vi "3_dynamic_friction_main.vi"() -> ()   [LabVIEW 2019]
uses:
  Shared VIs/ENPID/PID_Settings.ctl
  Shared VIs/ENPID/Gains.ctl
  Shared VIs/ENPID/NonLinearGainParams.ctl
  Shared VIs/ENPID/NonLinearGain.ctl
  Shared VIs/ENPID/DPartVariable.ctl
  Shared VIs/ENPID/VelocityEstimate.ctl
  Shared VIs/ENPID/OutputRange.ctl
  Shared VIs/TypeDef_TDMS_States.ctl
  <vilib>/myRIO/Common/Instrument Driver Framework/myRIO v1.0/Encoder/typedefs/Encoder Signal Mode.ctl
  Shared VIs/ModelSpecific/ETHMikeModel.ctl
  Shared VIs/ModelSpecific/ReadOnlyGlobalActions.ctl
  <vilib>/myRIO/Instrument Drivers/Onboard IO/AI/typedefs/AI Reference.ctl
  <vilib>/myRIO/Common/Instrument Driver Framework/Utilities/typedefs/myRIO Generic Hardware Reference.ctl
  <vilib>/myRIO/Common/Instrument Driver Framework/Utilities/typedefs/Hardware Version Enum.ctl
  <vilib>/myRIO/Common/Instrument Driver Framework/Utilities/typedefs/myRIO v1.0 Reference.ctl
  <vilib>/myRIO/Common/Instrument Driver Framework/Utilities/typedefs/Generic FPGA Reference.ctl
  <vilib>/myRIO/Common/Instrument Driver Framework/myRIO v1.0/AI/typedefs/AI Channels List.ctl
  <vilib>/myRIO/Common/Instrument Driver Framework/myRIO v1.0/AI/typedefs/AI Channels Enum.ctl
  <vilib>/myRIO/Common/Instrument Driver Framework/Utilities/typedefs/Analog Scaling Constants List.ctl
  <vilib>/myRIO/Common/Instrument Driver Framework/Utilities/typedefs/Analog Scaling Constants.ctl
  <vilib>/userDefined/High Color/nirio_resource_hc.ctl
  <vilib>/myRIO/Instrument Drivers/Onboard IO/AO/typedefs/AO Reference.ctl
  <vilib>/myRIO/Common/Instrument Driver Framework/myRIO v1.0/AO/typedefs/AO Channels List.ctl
  <vilib>/myRIO/Common/Instrument Driver Framework/myRIO v1.0/AO/typedefs/AO Channels Enum.ctl
  <vilib>/Platform/TimedLoop/XDataNode/timing_clust.ctl
  <vilib>/Platform/TimedLoop/XDataNode/nitl_modes.ctl
  <vilib>/Platform/TimedLoop/XDataNode/wakeup.ctl
  <vilib>/Analysis/3filter.llb/Filter Passband Type.ctl
  <vilib>/myRIO/Common/Instrument Driver Framework/myRIO v1.0/AI/vis/myRIO v1.1 Open AI.vi
  <vilib>/myRIO/Common/Instrument Driver Framework/myRIO v1.0/AO/vis/myRIO v1.1 Open AO.vi
  <vilib>/myRIO/Common/Instrument Driver Framework/Utilities/vis/Validate Channels.vi
  <vilib>/myRIO/Common/Instrument Driver Framework/myRIO v1.0/AI/vis/myRIO v1.0 Reserve AI.vi
  <vilib>/myRIO/Common/Instrument Driver Framework/myRIO v1.0/AO/vis/myRIO v1.0 Reserve AO.vi
  <vilib>/myRIO/Common/Instrument Driver Framework/myRIO v1.0/AI/vis/myRIO v1.0 Close AI.vi
  <vilib>/myRIO/Common/Instrument Driver Framework/myRIO v1.0/AO/vis/myRIO v1.0 Close AO.vi
  <vilib>/myRIO/Common/Instrument Driver Framework/myRIO v1.0/Encoder/vis/myRIO v1.0 Close Encoder.vi
  <vilib>/myRIO/Common/Instrument Driver Framework/myRIO v1.0/AI/vis/myRIO v1.0 Build MUX Configuration AI.vi
  <vilib>/myRIO/Common/Instrument Driver Framework/myRIO v1.0/Resource Manager/vis/myRIO v1.0 Reserve Channel List.vi
  <vilib>/myRIO/Common/Instrument Driver Framework/myRIO v1.0/AO/vis/myRIO v1.0 Build MUX Configuration AO.vi
  <vilib>/myRIO/Common/Instrument Driver Framework/myRIO v1.0/AI/vis/myRIO v1.0 Unreserve AI.vi
  <vilib>/myRIO/Common/Instrument Driver Framework/myRIO v1.0/AO/vis/myRIO v1.0 Unreserve AO.vi
  <vilib>/myRIO/Common/Instrument Driver Framework/myRIO v1.0/Encoder/vis/myRIO v1.0 Unreserve Encoder.vi
  <vilib>/myRIO/Common/Instrument Driver Framework/myRIO v1.0/Resource Manager/vis/myRIO v1.0 Reserve Channel.vi
  <vilib>/myRIO/Common/Instrument Driver Framework/myRIO v1.0/Resource Manager/vis/myRIO v1.0 Unreserve Channel.vi
  <vilib>/myRIO/Common/Instrument Driver Framework/myRIO v1.0/Resource Manager/vis/myRIO v1.0 Unreserve Channel List.vi
  <vilib>/myRIO/Common/Instrument Driver Framework/myRIO v1.0/Encoder/vis/myRIO v1.0 Build MUX Configuration Encoder.vi
  <vilib>/myRIO/Common/Instrument Driver Framework/myRIO v1.0/Resource Manager/vis/myRIO v1.0 Build Mutex Name.vi
  <vilib>/myRIO/Common/Instrument Driver Framework/myRIO v1.0/Resource Manager/vis/myRIO v1.0 Create Configuration List.vi
  <vilib>/Utility/VariantDataType/GetNumericInfo.vi
  <vilib>/Utility/error.llb/Error Cluster From Error Code.vi
  <vilib>/myRIO/Common/Instrument Driver Framework/myRIO v1.0/myRIO v1.1 Open.vi
  <vilib>/myRIO/Common/Instrument Driver Framework/myRIO v1.0/AO/vis/myRIO v1.0 Get Scaling Constants AO.vi
  <vilib>/myRIO/Common/Instrument Driver Framework/Utilities/vis/IO Manager.vi
  <vilib>/myRIO/Common/Instrument Driver Framework/Utilities/vis/Configuration Manager.vi
  <vilib>/myRIO/Common/Instrument Driver Framework/myRIO v1.0/myRIO v1.0 Close.vi
  <vilib>/myRIO/Common/Instrument Driver Framework/myRIO v1.0/AO/vis/myRIO v1.0 Write AO.vi
  <vilib>/myRIO/Common/Instrument Driver Framework/myRIO v1.0/AI/vis/myRIO v1.0 Get Scaling Constants AI.vi
  <vilib>/myRIO/Common/Instrument Driver Framework/myRIO v1.0/AI/vis/myRIO v1.0 Read AI.vi
  <vilib>/myRIO/Common/Instrument Driver Framework/myRIO v1.0/Encoder/vis/myRIO v1.0 Read Encoder.vi
  <vilib>/myRIO/Common/Instrument Driver Framework/myRIO v1.0/Encoder/vis/myRIO v1.0 Enable Encoder.vi
  <vilib>/myRIO/Common/Instrument Driver Framework/myRIO v1.0/Encoder/vis/myRIO v1.0 Shutdown Encoder.vi
  <vilib>/myRIO/Common/Instrument Driver Framework/myRIO v1.0/Resource Manager/vis/myRIO v1.0 Configure IO.vi
  <vilib>/myRIO/Instrument Drivers/Onboard IO/AO/vis/myRIO AO Open.xnode
  <vilib>/myRIO/Instrument Drivers/Onboard IO/AI/vis/myRIO AI Open.xnode
  <vilib>/Platform/TimedLoop/XDataNode/XDataNode.xnode
  <vilib>/Platform/TimedLoop/XDataNode/XDNodeRunTimeDep.lvlib
  <vilib>/addons/control/pid/NI_PID_pid.lvlib
  <vilib>/myRIO/Instrument Drivers/Onboard IO/AO/AO.lvlib
  <vilib>/myRIO/Instrument Drivers/Onboard IO/Encoder/Encoder.lvlib
  <vilib>/myRIO/Instrument Drivers/Onboard IO/AI/AI.lvlib
  <vilib>/Analysis/NI_AALBase.lvlib
  <vilib>/ptbypt/NI_PtbyPt.lvlib
panel:
  out "u_direct":dbl
  out "ud":dbl
  out "ui":dbl
  out "up":dbl
  out "u":dbl
  out "Running":dbl
  in  "Ramp Distance (°)":dbl
  in  "TDMS Storage File Input":string
  out "TDMS States":T1
  in  "PID Settings":T2={"Gains"={"K(e)"=0.0, "Kp"=0.800000011920929, "Ki"=0.0, "Kd"=0.003000000026077032}, "Non-linear gain"={"Non-linear gain P"=enum."off", "Non-linear gain I"=enum."off", "Non-linear gain D"=enum."off"}, "D-Part variable"=enum."process variable", "Velocity estimate dy/dt"=enum."external", "Anti reset windup"=TRUE, "I-Part error band"=inf, "Output range"={"output high"=0.0, "output low"=0.0}}
  in  "STOP":bool
  out "Current [A]":dbl
  out "Current Setpoint [A]":dbl
  out "Velocity [deg/s]":dbl
  out "Position [deg]":dbl
  out "Position Setpoint [deg]":dbl
  in  "Save data?":bool
  in  "Run":bool
  out "Position Setpoint Chart":dbl(graph)
  out "Time (s)":dbl
  out "Current Setpoint Chart":dbl(graph)
  out "Velocity Chart":dbl(graph)
  out "Position Chart":dbl(graph)
  in  "Ramp Duration (s)":dbl
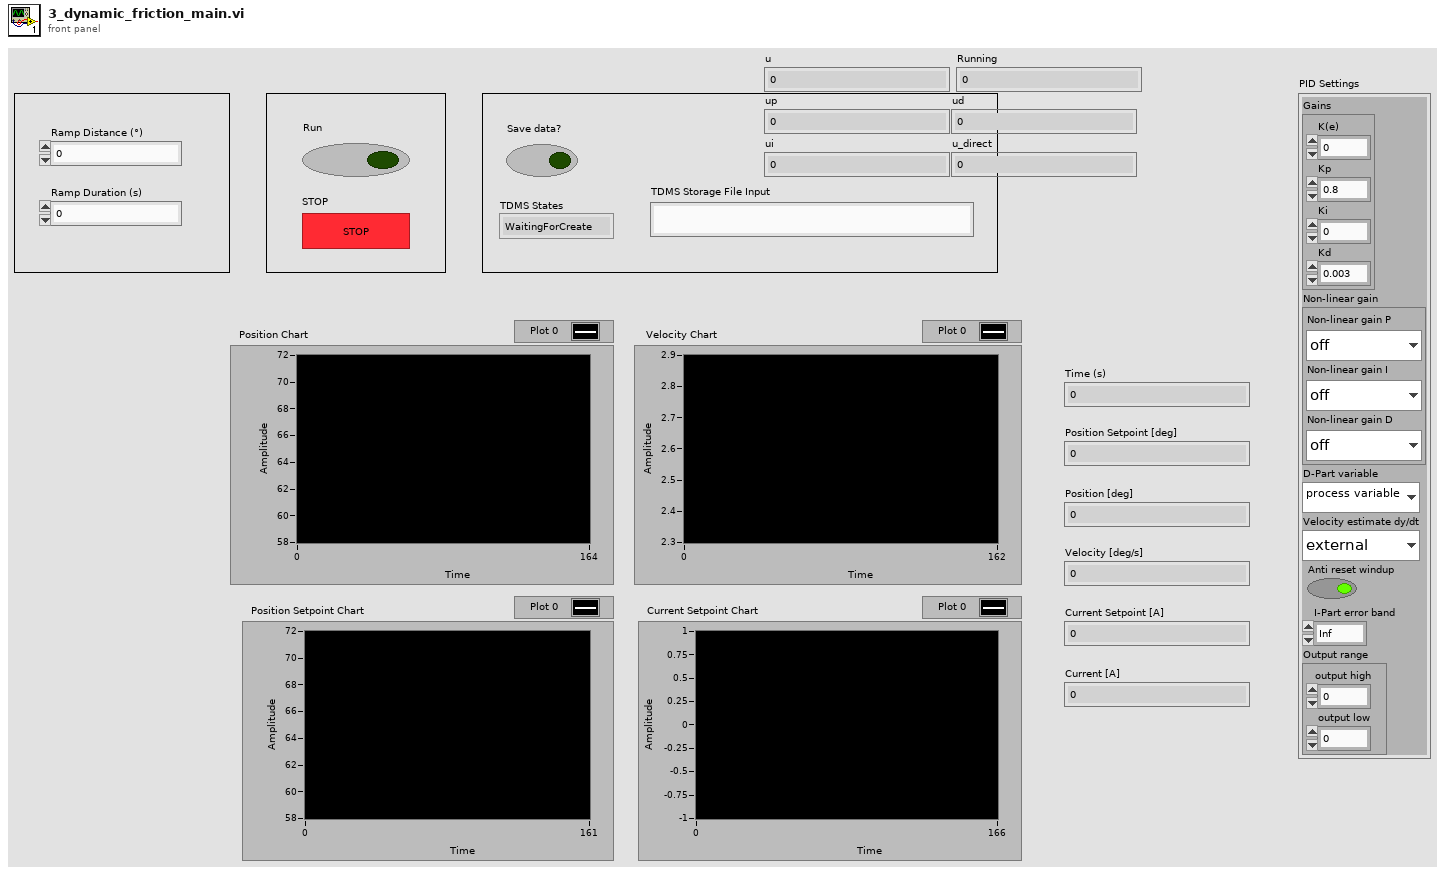
[diagram p1: front panel]
types:
  T1 = typedef "TypeDef_TDMS_States.ctl" = enum16{"WaitingForCreate", "Create", "Buffering", "Flushing", "Write", "Close"}
  T2 = typedef "PID_Settings.ctl" = cluster{"Gains":T3, "Non-linear gain":T4, "D-Part variable":T6, "Velocity estimate dy/dt":T7, "Anti reset windup":bool, "I-Part error band":dbl, "Output range":T8}
  T3 = typedef "Gains.ctl" = cluster{"K(e)":dbl, "Kp":dbl, "Ki":dbl, "Kd":dbl}
  T4 = typedef "NonLinearGainParams.ctl" = cluster{"Non-linear gain P":T5, "Non-linear gain I":T5, "Non-linear gain D":T5}
  T5 = typedef "NonLinearGain.ctl" = enum16{"exponential", "quadratic", "off"}
  T6 = typedef "DPartVariable.ctl" = enum16{"error", "process variable"}
  T7 = typedef "VelocityEstimate.ctl" = enum16{"derivative", "external"}
  T8 = typedef "OutputRange.ctl" = cluster{"output high":dbl, "output low":dbl}
  T9 = typedef "nirio_resource_hc.ctl" = tag
  T10 = typedef "Hardware Version Enum.ctl" = enum16{"Unknown", "myRIO-1900", "myRIO-1950", "roboRIO", "NI ELVIS RIO CM", "ELVIS III"}
  T11 = enum16{"open", "open or create", "create or replace", "create", "open (read-only)"}
  T12 = typedef "XDNodeRunTimeDep.lvlib/timing_clust.ctl" = cluster{"Expected End [f-1]":u64, "Actual End [f-1]":u64, "Finished Late? [f-1]":bool, "Expected End [i-1]":u64, "Actual End [i-1]":u64, "Finished Late? [i-1]":bool, "Expected Start [i]":u64, "Actual Start [i]":u64, "Expected Start [f]":u64, "Actual Start [f]":u64, "Source Name":string, "Structure Name":string, "Period":i64, "Deadline":i64, "Offset":i64, "Start":i64, "Priority":i32, "Timeout":i32, "Mode":T13, "Wakeup Reason":T14, "Error":errorcluster, "Source Type":string, "Secondary Source Type":string, "Global End Time":u64, "Global Start Time":u64, "Frame Duration":u64, "Iteration Duration":u64, "Assigned CPU":i32, "I/O Scan Engine Mode":u32}
  T13 = typedef "XDNodeRunTimeDep.lvlib/nitl_modes.ctl" = enum32{"No Change", "Process missed periods, maintain original phase", "Discard missed periods, maintain original phase", "Process missed periods, ignore original phase", "Discard missed periods, ignore original phase"}
  T14 = typedef "XDNodeRunTimeDep.lvlib/wakeup.ctl" = enum32{"Normal", "Aborted", "Asynchronous wakeup", "Timing source error", "Timed loop error", "Timeout"}
  T15 = typedef "NI_AALBase.lvlib/Filter Passband Type.ctl" = enum32{"Lowpass", "Highpass", "Bandpass", "Bandstop"}
  T16 = typedef "ReadOnlyGlobalActions.ctl" = enum16{"Initialize", "Read", "Write"}
  T17 = typedef "ETHMikeModel.ctl" = enum16{"ETH Mike #1", "ETH Mike #2", "ETH Mike #3", "ETH Mike #4", "ETH MIKE #5"}
  T18 = typedef "Encoder Signal Mode.ctl" = enum16{"Quadrature phase signal", "Step and direction signal"}
  T19 = typedef "AO.lvlib/AO Reference.ctl" = cluster{"myRIO Reference":T20, "AO Channel List":T23, "AO Scaling Constant List":T25}
  T20 = typedef "myRIO Generic Hardware Reference.ctl" = cluster{"myRIO Model":T10, "myRIO Hardware Reference":T21}
  T21 = typedef "myRIO v1.0 Reference.ctl" = cluster{"Generic FPGA Reference":T22, "Allow multiple opens":bool}
  T22 = typedef "Generic FPGA Reference.ctl" = refnum<k20>
  T23 = typedef "AO Channels List.ctl" = T24[]
  T24 = typedef "AO Channels Enum.ctl" = enum16{"Not Connected", "AudioOut/Left", "AudioOut/Right", "C/AO0", "C/AO1", "A/AO0", "A/AO1", "B/AO0", "B/AO1"}
  T25 = typedef "Analog Scaling Constants List.ctl" = T26[]
  T26 = typedef "Analog Scaling Constants.ctl" = cluster{"LSB Weight (Volts)":dbl, "Offset (Volts)":dbl, "Signed?":bool}
  T27 = typedef "AI.lvlib/AI Reference.ctl" = cluster{"myRIO Reference":T20, "AI Channels List":T28, "AI Scaling Constants List":T25}
  T28 = typedef "AI Channels List.ctl" = T29[]
  T29 = typedef "AI Channels Enum.ctl" = enum16{"Not Connected", "AudioIn/Left", "AudioIn/Right", "C/AI0", "C/AI1", "A/AI0", "A/AI1", "A/AI2", "A/AI3", "A/AI4", "A/AI5", "A/AI6", "A/AI7", "B/AI0", "B/AI1", "B/AI2", "B/AI3", "B/AI4", "B/AI5", "B/AI6", "B/AI7", "AI/AI0", "AI/AI1", "AI/AI2", "AI/AI3", "A/AI0 (DIFF)", "A/AI1 (DIFF)", "A/AI2 (DIFF)", "A/AI3 (DIFF)", "B/AI0 (DIFF)", "B/AI1 (DIFF)", "B/AI2 (DIFF)", "B/AI3 (DIFF)"}
  T30 = typedef "Encoder.lvlib/Encoder Reference.ctl" = cluster{"myRIO Reference":T20, "Encoder Channels Enum":T31}
  T31 = typedef "Encoder Channels Enum.ctl" = enum16{"Not Connected", "C/ENC0", "C/ENC1", "A/ENC", "A/ENC0", "A/ENC1", "A/ENC2", "A/ENC3", "A/ENC4", "A/ENC5", "A/ENC6", "A/ENC7", "A/ENC8", "A/ENC9", "B/ENC", "B/ENC0", "B/ENC1", "B/ENC2", "B/ENC3", "B/ENC4", "B/ENC5", "B/ENC6", "B/ENC7", "B/ENC8", "B/ENC9", "DIO/ENC0", "DIO/ENC1", "DIO/ENC2", "DIO/ENC3", "DIO/ENC4"}
  T32 = typedef "TypeDefTachometerParam.ctl" = cluster{"Offset [V]":dbl, "Gain [deg/sV]":dbl}
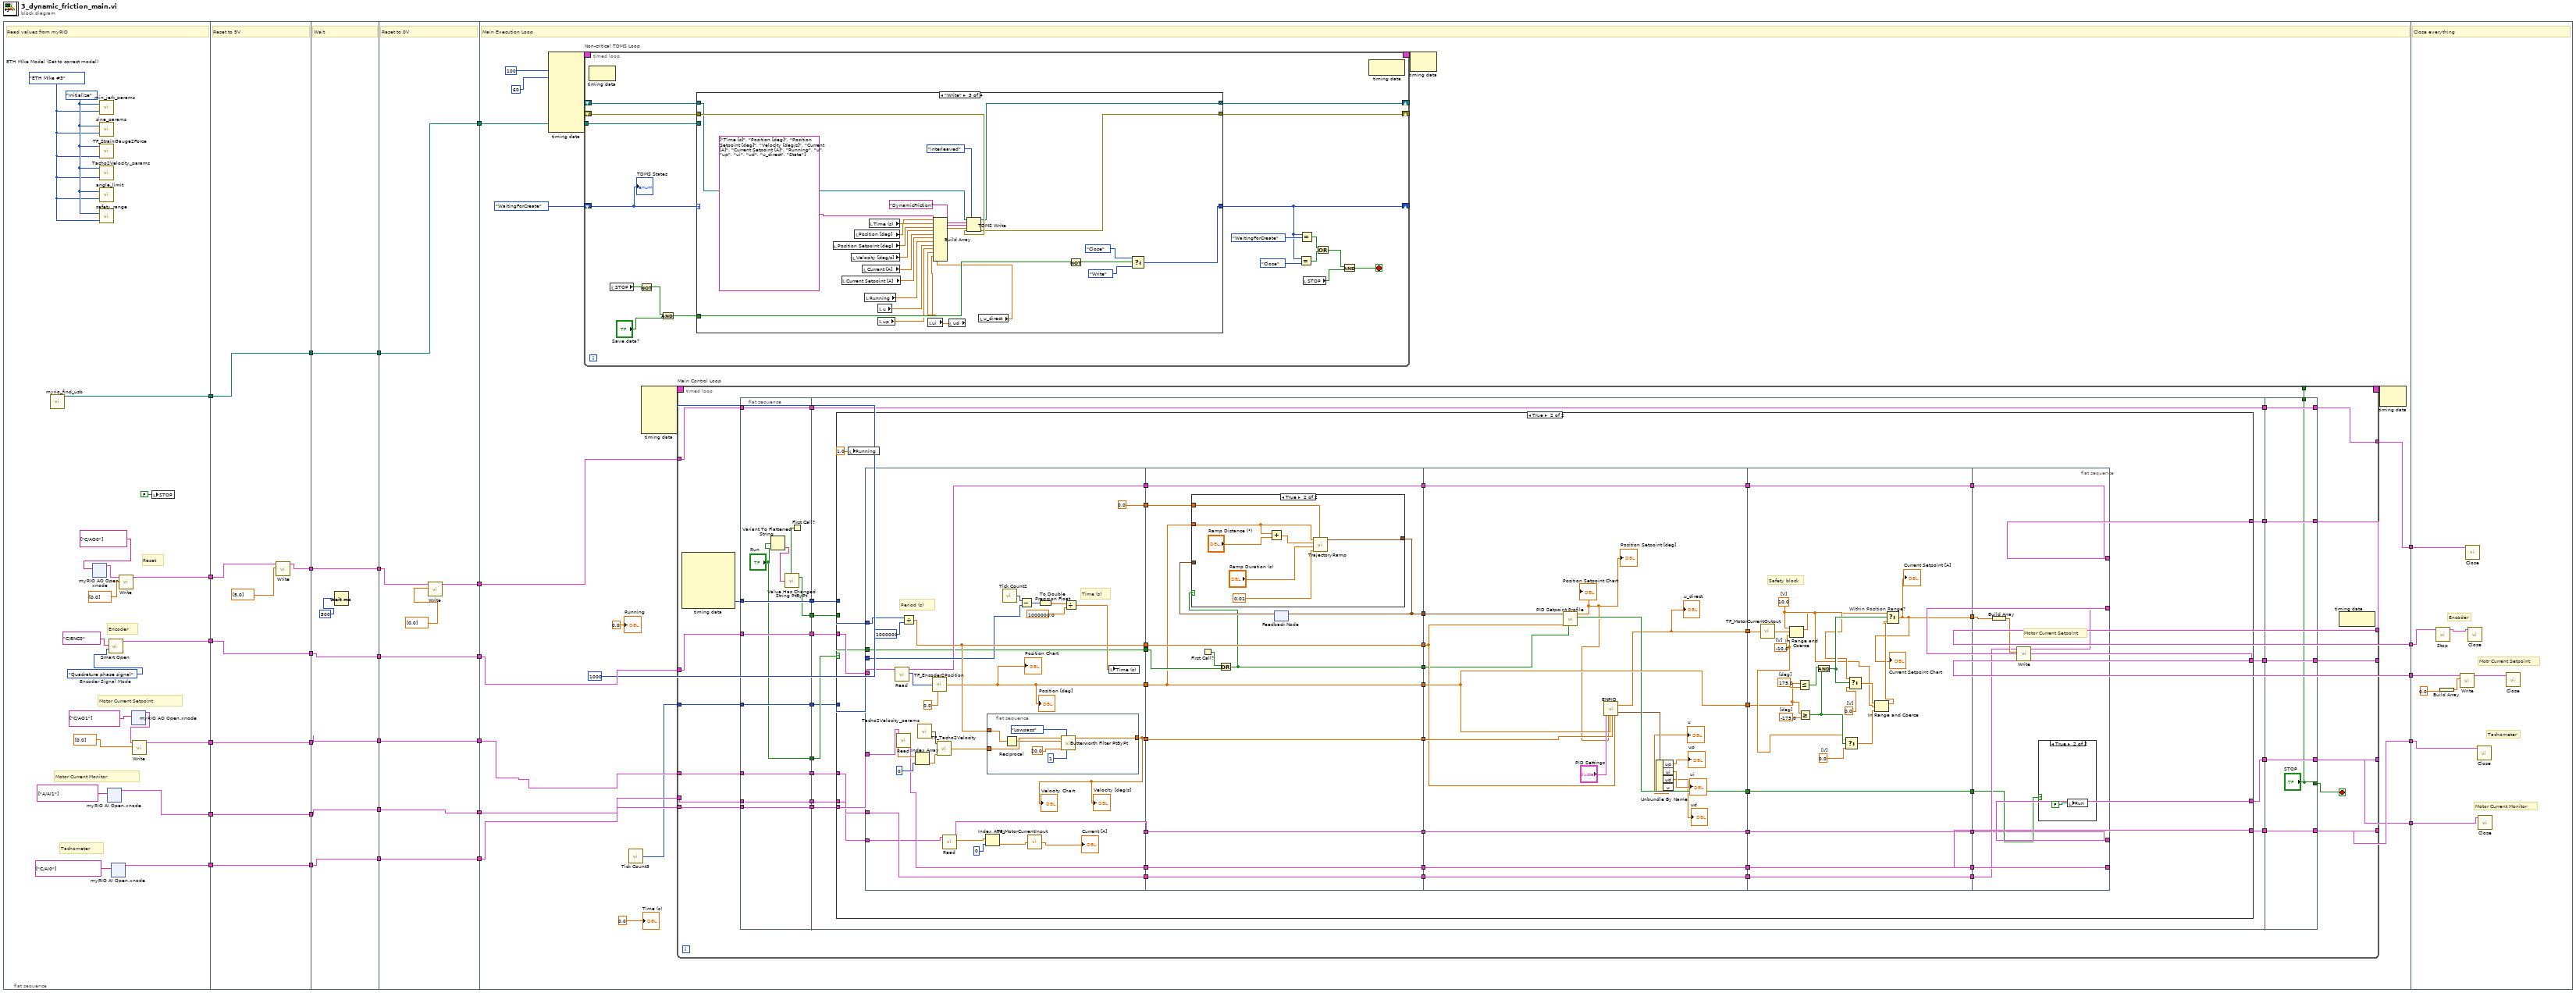
[diagram p0: block diagram]
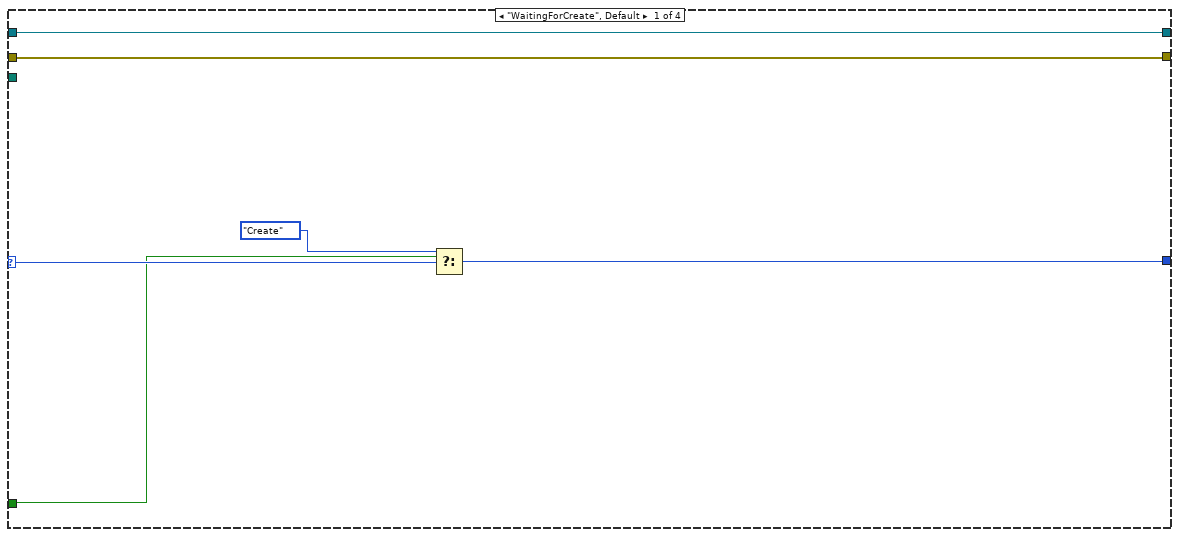
[diagram p2: hidden frame]
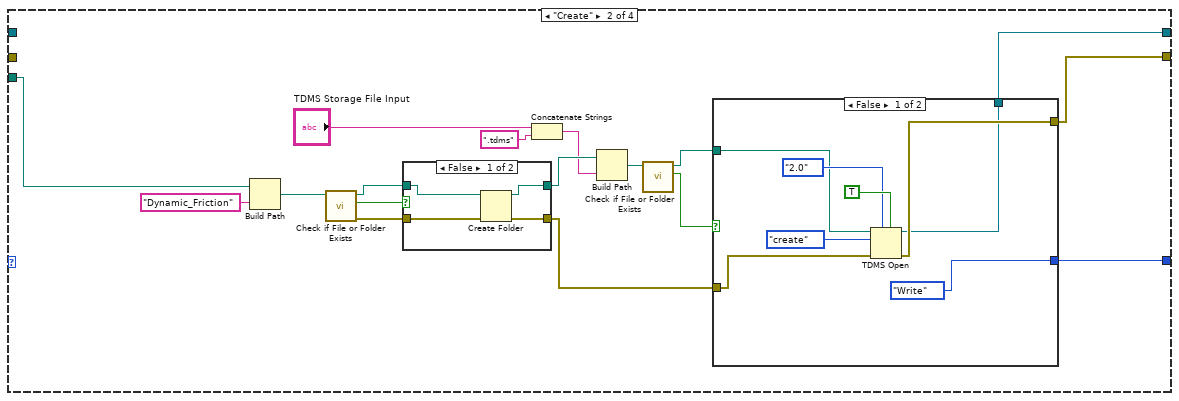
[diagram p3: hidden frame]
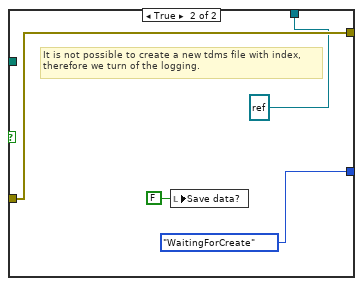
[diagram p4: hidden frame]
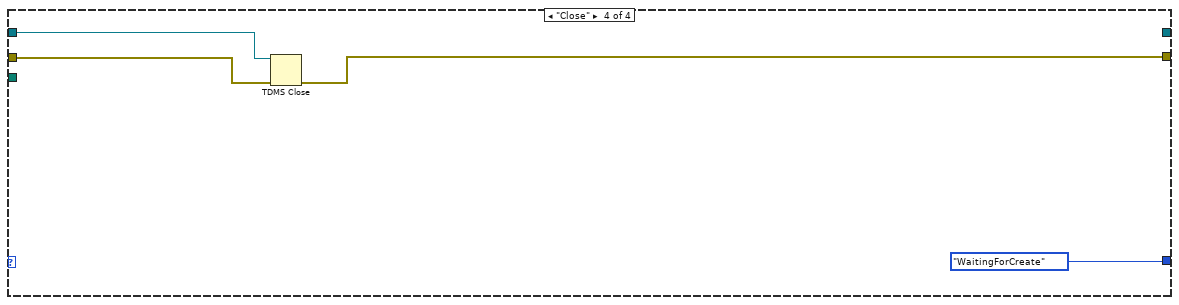
[diagram p6: hidden frame]
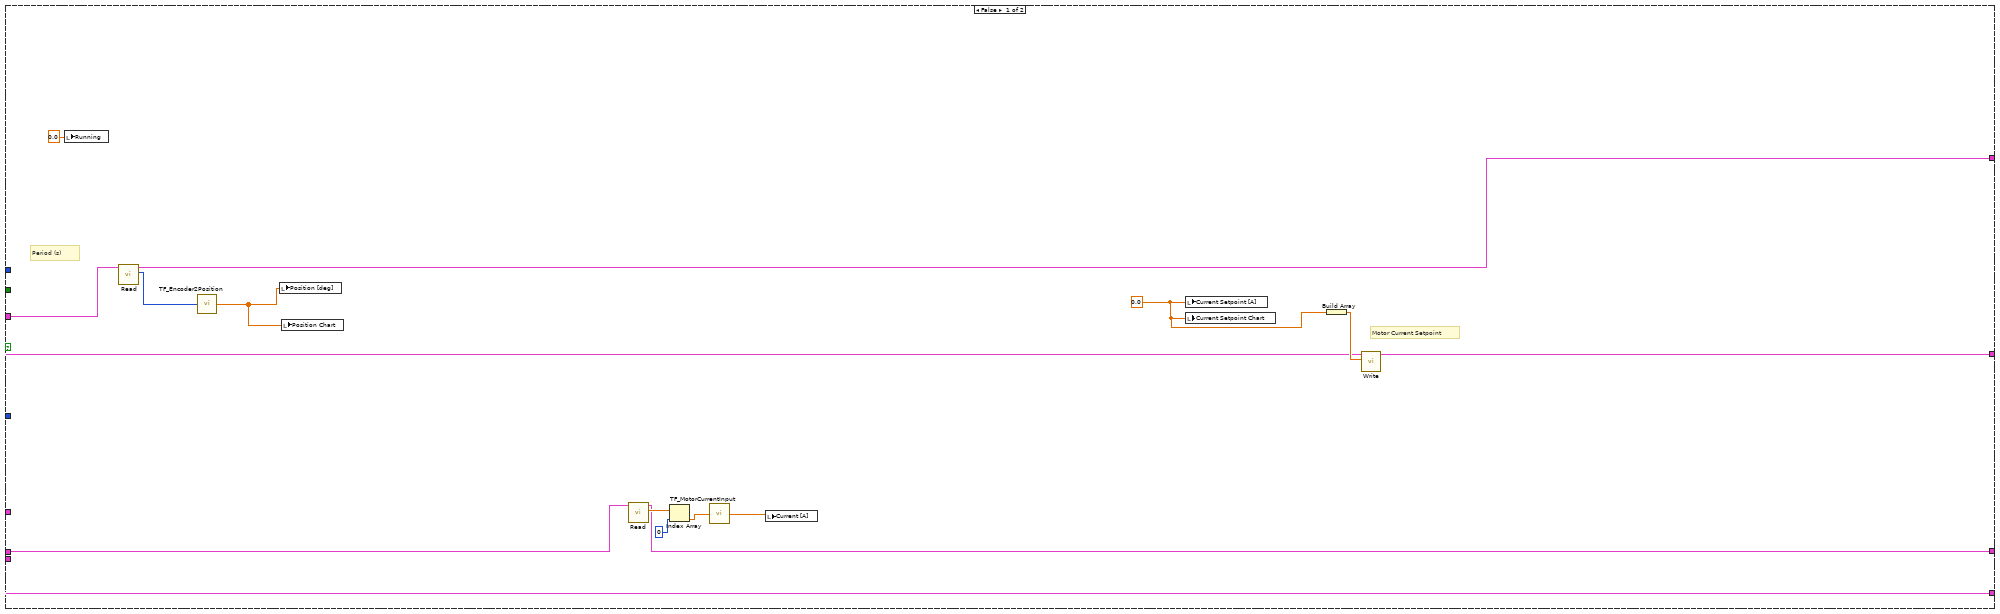
[diagram p7: hidden frame]
diagram:
  n1 = flat-sequence {
    tunnel: [w45] -> w29
    tunnel: [w42] -> w26
    tunnel: [w38] -> w25
    tunnel: [w36] -> w24
    tunnel: [w34] -> w23
    tunnel: [w33] -> w1
    tunnel: w29 -> [w127]
    tunnel: [w126] -> w28
    tunnel: w26 -> [w125]
    tunnel: w25 -> [w124]
    tunnel: w24 -> [w123]
    tunnel: w23 -> [w122]
    tunnel: [w125] -> w22
    tunnel: [w124] -> w18
    tunnel: [w123] -> w14
    tunnel: [w122] -> w13
    tunnel: [w121] -> w2
    tunnel: w1 -> [w121]
    tunnel: w28 -> [w135]
    tunnel: [w135] -> w27
    tunnel: w22 -> [w133]
    tunnel: [w133] -> w21
    tunnel: [w132] -> w19
    tunnel: w18 -> [w132]
    tunnel: [w131] -> w15
    tunnel: w14 -> [w131]
    tunnel: w13 -> [w130]
    tunnel: [w130] -> w11
    tunnel: [w129] -> w3
    tunnel: w2 -> [w129]
    tunnel: w27 -> [w142]
    tunnel: w21 -> [w141]
    tunnel: [w141] -> w20
    tunnel: w19 -> [w140]
    tunnel: [w140] -> w17
    tunnel: [w139] -> w16
    tunnel: w15 -> [w139]
    tunnel: [w138] -> w12
    tunnel: w11 -> [w138]
    tunnel: [w137] -> w7
    tunnel: [w136] -> w4
    tunnel: w3 -> [w136]
    tunnel: w20 -> [w165]
    tunnel: w17 -> [w163]
    tunnel: w16 -> [w160]
    tunnel: w12 -> [w164]
    tunnel: [w162] -> w10
    tunnel: [w161] -> w9
    tunnel: [w159] -> w8
    tunnel: w7 -> [w154]
    tunnel: [w155] -> w6
    tunnel: [w145] -> w5
    tunnel: w4 -> [w146]
    tunnel: w10 -> [w497]
    tunnel: w9 -> [w496]
    tunnel: w8 -> [w495]
    tunnel: w6 -> [w493]
    tunnel: w5 -> [w494]
    frame #0 {
      w32 = ReadOnlyGlobalActions."Initialize" ("Action (Read)")
      w31 = ETHMikeModel."ETH Mike #3"  # ETH Mike Model (Set to correct model)
      w43 = Encoder_Signal_Mode."Quadrature phase signal"  # Encoder Signal Mode
      # "Tachometer"
      # "Motor Current Monitor"
      # "Motor Current Setpoint"
      # "Reset"
      # "Encoder"
      # "Read values from myRIO"
      n2 = call "myrio_find_usb.vi"() -> ("Largest USB Partition Path"=w33:path)  [unwired: 9 in, 2 out]
      n3 = xnode "myRIO AO Open.xnode"("Channel Names"=tag[] ["C/AO0"]) -> ("AO Ref Out"=w47:T19)  [unwired: 2 in, 1 out]
      n4 = call "min_jerk_params.vi"("Action (Read)"=w32, "ETH Mike Model"=w31) -> ()  [unwired: 17 in, 1 out]
      n5 = call "sine_params.vi"("Action (Read)"=w32, "ETH Mike Model"=w31) -> ()  [unwired: 17 in, 1 out]
      n6 = call "TF_StrainGauge2Force.vi"("Action (Read)"=w32, "ETH Mike Model"=w31) -> ()  [unwired: 3 in, 1 out]
      n7 = call "Tacho2Velocity_params.vi"("Action (Read)"=w32, "ETH Mike Model"=w31) -> ()  [unwired: 3 in, 1 out]
      n8 = call "angle_limit.vi"("ETH Mike Model"=w31, "Action (Read)"=w32) -> ()  [unwired: 1 out]
      n9 = call "safety_range.vi"("ETH Mike Model"=w31, "Action (Read)"=w32) -> ()  [unwired: 1 out]
      n10 = xnode "myRIO AI Open.xnode"("Channel Names"=tag[] ["A/AI1"]) -> ("AI Ref Out"=w36:T27)  [unwired: 2 in, 1 out]
      n11 = call <vilib>:"Smart Open.vi"("Encoder Signal Mode"=w43, "Channel Name"=tag "C/ENC0") -> ("Encoder Ref Out"=w42:T30)  [unwired: 8 in, 1 out]
      n12 = xnode "myRIO AI Open.xnode"("Channel Names"=tag[] ["C/AI0"]) -> ("AI Ref Out"=w34:T27)  [unwired: 2 in, 1 out]
      n13 = call <vilib>:"Write.vi"("Values"=dbl[] [0.0], "AO Ref In"=w47) -> ("AO Ref Out"=w45:T19)  [unwired: 7 in, 1 out]
      n14 = xnode "myRIO AO Open.xnode"("Channel Names"=tag[] ["C/AO1"]) -> ("AO Ref Out"=w40:T19)  [unwired: 2 in, 1 out]
      n15 = call <vilib>:"Write.vi"("Values"=dbl[] [0.0], "AO Ref In"=w40) -> ("AO Ref Out"=w38:T19)  [unwired: 7 in, 1 out]
      n16 = local write "STOP"(FALSE ("STOP")) -> ()
    }
    frame #1 {
      # "Reset to 5V"
      n17 = call <vilib>:"Write.vi"("Values"=dbl[] [5.0], "AO Ref In"=w127) -> ("AO Ref Out"=w126:T19)  [unwired: 7 in, 1 out]
    }
    frame #2 {
      # "Wait"
      n18 = Wait (ms)(milliseconds to wait=500) -> ()  [unwired: 1 out]
    }
    frame #3 {
      # "Reset to 0V"
      n19 = call <vilib>:"Write.vi"("Values"=dbl[] [0.0], "AO Ref In"=w142) -> ("AO Ref Out"=w137:T19)  [unwired: 7 in, 1 out]
    }
    frame #4 {
      # "Main Execution Loop"
      n20 = node-c288(100, 60) -> (w151:T12)  [unwired: 8 in]
      n21 = timed-loop "Non-critical TDMS Loop" {
        timing: w151 -> [_]
        timing-out: [_] -> w150
        shift-right: [w171] -> _
        shift-left: TypeDef_TDMS_States."WaitingForCreate" ("TDMS States") -> [w178]
        tunnel: w146 -> [w183]
        shift-right: [w182] -> _
        shift-left: _ -> [w179]
        shift-right: [w181] -> _
        shift-left: _ -> [w180]
        stop <- w166 stop-if-true
        n22 = node-c288() -> ()  [unwired: 1 in, 1 out]
        n23 = local read "STOP"() -> (w177:bool)
        n24 = Not(x=w177) -> (.not. x?=w175:bool)
        n25 = And(x=w175, y="Save data?") -> (x .and. y?=w174:bool)
        n26 = case shown="\"Write\"" w178 {
          selector: w178 -> [w188 _ _ _]
          tunnel: [w187 w190 w232 TypeDef_TDMS_States."WaitingForCreate" ("TDMS States")] -> w171
          tunnel: w183 -> [_ w196 _ _]
          tunnel: [w184 w191 w231 _] -> w182
          tunnel: [w185 w192 w237 w251] -> w181
          tunnel: w180 -> [w185 _ w239 w252]
          tunnel: w179 -> [w184 _ w238 w253]
          tunnel: w174 -> [w186 _ w233 _]
          frame "WaitingForCreate", Default {
            n27 = Select(t=TypeDef_TDMS_States."Create" ("TDMS States"), s=w186, f=w188) -> (s? t:f=w187:T1)
          }
          frame "Create" {
            n28 = Build Path(base path=w196, name or relative path="Dynamic_Friction") -> (appended path=w198:path)
            n29 = call <vilib>:"Check if File or Folder Exists.vi"("path"=w198) -> ("error out"=w204:errorcluster, "file or folder exists?"=w206:bool, "dup path"=w205:path)  [unwired: 8 in]
            n30 = case shown="False" w206 {
              tunnel: w205 -> [w222 w223]
              tunnel: [w221 w224] -> w193
              tunnel: w204 -> [w220 w224]
              tunnel: [w219 w223] -> w203
              frame False {
                n31 = Create Folder(path (use dialog)=w222, error in=w220) -> (created path=w219:path, error out=w221:errorcluster)  [unwired: 1 in, 1 out]
              }
              frame True {
              }
            }
            n32 = Concatenate Strings("TDMS Storage File Input", ".tdms") -> (w200:string)
            n33 = Build Path(base path=w203, name or relative path=w200) -> (appended path=w199:path)
            n34 = call <vilib>:"Check if File or Folder Exists.vi"("path"=w199) -> ("file or folder exists?"=w195:bool, "dup path"=w194:path)  [unwired: 8 in, 1 out]
            n35 = case shown="False" w195 {
              tunnel: w194 -> [w211 _]
              tunnel: w193 -> [w210 w218]
              tunnel: [w209 w218] -> w192
              tunnel: [w208 refnum<k34> refnum ("tdms file out")] -> w191
              tunnel: [TypeDef_TDMS_States."Write" ("TDMS States") TypeDef_TDMS_States."WaitingForCreate" ("TDMS States")] -> w190
              frame False {
                n36 = TDMS Open(5:TRUE, 7:enum16{"1.0", "2.0"}."2.0" ("file format version (2.0)"), 8:w210, 10:T11."create" ("operation (0:open)"), 11:w211) -> (0:w209:errorcluster, 3:w208:refnum<k34>)  [unwired: 2 in]
              }
              frame True {
                # "It is not possible to create a new tdms file with index,\ntherefore we turn of the logging."
                n37 = local write "Save data?"(FALSE ("Save data?")) -> ()
              }
            }
          }
          frame "Write" {
            n38 = local read "Position Setpoint [deg]"() -> (w246:dbl)
            n39 = local read "Current Setpoint [A]"() -> (w243:dbl)
            n40 = local read "Velocity [deg/s]"() -> (w245:dbl)
            n41 = local read "Position [deg]"() -> (w247:dbl)
            n42 = local read "Current [A]"() -> (w244:dbl)
            n43 = local read "Running"() -> (w230:dbl)
            n44 = local read "Time (s)"() -> (w242:dbl)
            n45 = local read "u"() -> (w229:dbl)
            n46 = local read "up"() -> (w228:dbl)
            n47 = local read "ui"() -> (w227:dbl)
            n48 = local read "ud"() -> (w226:dbl)
            n49 = local read "u_direct"() -> (w225:dbl)
            n50 = Build Array(w242, w247, w246, w245, w244, w243, w230, w229, w228, w227, w226, w225) -> (w241:dbl[])
            n51 = TDMS Write(0:w238, 1:enum16{"decimated", "interleaved"}."interleaved" ("data layout (0:decimated)"), 5:"DynamicFriction" ("group name in (Untitled)"), 7:string[] ["Time [s]", "Position [deg]", "Position Setpoint [deg]", "Velocity [deg/s]", "Current [A]", "Current Setpoint [A]", "Running", "u", "up", "ui", "ud", "u_direct", "State"], 9:w241, 11:w239) -> (4:w231:refnum<k34>, 15:w237:errorcluster)  [unwired: 2 out]
            n52 = Not(x=w233) -> (.not. x?=w236:bool)
            n53 = Select(t=TypeDef_TDMS_States."Close" ("TDMS States"), s=w236, f=TypeDef_TDMS_States."Write" ("TDMS States")) -> (s? t:f=w232:T1)
          }
          frame "Close" {
            n54 = TDMS Close(8:w252, 11:w253) -> (0:w251:errorcluster)  [unwired: 1 out]
          }
        }
        n55 = Equal?(x=w171, y=TypeDef_TDMS_States."Close" ("TDMS States")) -> (x = y?=w169:bool)
        n56 = Equal?(x=w171, y=TypeDef_TDMS_States."WaitingForCreate" ("TDMS States")) -> (x = y?=w170:bool)
        n57 = local read "STOP"() -> (w167:bool)
        n58 = Or(x=w170, y=w169) -> (x .or. y?=w168:bool)
        n59 = And(x=w168, y=w167) -> (x .and. y?=w166:bool)
        n60 = node-c288() -> ()  [unwired: 1 in, 1 out]
        "TDMS States" <- w178
      }
      n61 = call "Tick Count3"() -> ("Tick Count(uSec)"=w153:u32)
      n62 = node-c288(1000) -> (w158:T12)  [unwired: 4 in]
      n63 = timed-loop "Main Control Loop" {
        timing: w158 -> [_]
        timing-out: [_] -> w157
        tunnel: w165 -> [w287]
        tunnel: w164 -> [w286]
        tunnel: w163 -> [w282]
        tunnel: [w285] -> w162
        tunnel: [w284] -> w161
        tunnel: w160 -> [w280]
        tunnel: [w283] -> w159
        tunnel: [w277] -> w155
        tunnel: w154 -> [w278]
        tunnel: w153 -> [w281]
        tunnel: [w279] -> w145
        tunnel: [w261] -> _
        stop <- w262 stop-if-true
        n64 = node-c288() -> (w288:i64)  [unwired: 1 in, 6 out]
        n65 = flat-sequence {
          tunnel: w278 -> [w293]
          tunnel: w280 -> [w294]
          tunnel: w281 -> [w295]
          tunnel: w282 -> [w296]
          tunnel: w286 -> [w297]
          tunnel: w287 -> [w298]
          tunnel: w288 -> [w299]
          tunnel: [w299] -> w271
          tunnel: [w298] -> w270
          tunnel: [w297] -> w269
          tunnel: [w296] -> w268
          tunnel: ["Run"] -> w267
          tunnel: [w295] -> w266
          tunnel: [w294] -> w265
          tunnel: [w289] -> w264
          tunnel: [w293] -> w263
          tunnel: [w309] -> w276
          tunnel: [w308] -> w275
          tunnel: [w307] -> w274
          tunnel: [w302] -> w273
          tunnel: [w300] -> w272
          tunnel: w271 -> [w312]
          tunnel: w270 -> [w311]
          tunnel: w269 -> [w310]
          tunnel: w268 -> [w306]
          tunnel: w267 -> [w305]
          tunnel: w266 -> [w304]
          tunnel: w265 -> [w303]
          tunnel: w264 -> [w301]
          tunnel: w263 -> [w300]
          tunnel: [w481] -> w277
          tunnel: [w482] -> w279
          tunnel: [w483] -> w283
          tunnel: [w484] -> w284
          tunnel: [w485] -> w285
          tunnel: w276 -> [w485]
          tunnel: w275 -> [w484]
          tunnel: w274 -> [w483]
          tunnel: w273 -> [w482]
          tunnel: w272 -> [w481]
          tunnel: ["STOP"] -> w262
          tunnel: ["STOP"] -> w261
          frame #0 {
            n66 = Variant To Flattened String(Variant="Run") -> (data string=w291:string)  [unwired: 1 out]
            n67 = First Call?() -> (First Call?: T/F=w292:bool)
            n68 = call "Value Has Changed String PtByPt.vi"("input data point"=w291, "initialize"=w292) -> ("has changed"=w289:bool)  [unwired: 1 out]
          }
          frame #1 {
            n69 = case shown="True" w305 {
              tunnel: w312 -> [_ w368]
              tunnel: w311 -> [w328 w367]
              tunnel: w310 -> [w314 w366]
              tunnel: [w315 w365] -> w309
              tunnel: [w327 w350] -> w308
              tunnel: [w314 w360] -> w307
              tunnel: w306 -> [w316 w359]
              tunnel: w301 -> [_ w356]
              tunnel: w304 -> [_ w355]
              tunnel: w303 -> [w321 w354]
              tunnel: [w320 w351] -> w302
              frame False {
                w317 = 0.0 ("Current Setpoint [A]")
                # "Motor Current Setpoint"
                # "Period (s)"
                n70 = local write "Running"(0.0 ("Running")) -> ()
                n71 = call <vilib>:"Read.vi"("Encoder Ref In"=w328) -> ("Counter Value"=w326:i32, "Encoder Ref Out"=w327:T30)  [unwired: 6 in, 3 out]
                n72 = call "TF_Encoder2Position.vi"("Counter Value"=w326) -> ("Position [deg]"=w325:dbl)  [unwired: 4 in]
                n73 = local write "Position [deg]"(w325) -> ()
                n74 = local write "Position Chart"(w325) -> ()
                n75 = call <vilib>:"Read.vi"("AI Ref In"=w321) -> ("Values"=w323:dbl[], "AI Ref Out"=w320:T27)  [unwired: 8 in, 1 out]
                n76 = Index Array(array=w323, index=0) -> (element=w322:dbl)
                n77 = call "TF_MotorCurrentInput.vi"("Motor Current Monitor Value [V]"=w322) -> ("Current [A]"=w319:dbl)
                n78 = local write "Current [A]"(w319) -> ()
                n79 = local write "Current Setpoint Chart"(w317) -> ()
                n80 = local write "Current Setpoint [A]"(w317) -> ()
                n81 = Build Array(w317) -> (w318:dbl[])
                n82 = call <vilib>:"Write.vi"("Values"=w318, "AO Ref In"=w316) -> ("AO Ref Out"=w315:T19)  [unwired: 7 in, 1 out]
              }
              frame True {
                n83 = local write "Running"(1.0 ("Running")) -> ()
                n84 = flat-sequence {
                  tunnel: w368 -> [w401]
                  tunnel: [w394] -> w347
                  tunnel: w367 -> [w400]
                  tunnel: [w376] -> w345
                  tunnel: w366 -> [w397]
                  tunnel: [w372] -> w343
                  tunnel: w355 -> [w392]
                  tunnel: [0.0] -> w341
                  tunnel: [w388] -> w340
                  tunnel: [w387] -> w338
                  tunnel: w359 -> [w386]
                  tunnel: [w386] -> w336
                  tunnel: w356 -> [w384]
                  tunnel: [w384] -> w334
                  tunnel: w354 -> [w378]
                  tunnel: [w377] -> w333
                  tunnel: w347 -> [w422]
                  tunnel: [w422] -> w346
                  tunnel: w345 -> [w410]
                  tunnel: [w410] -> w344
                  tunnel: w343 -> [w421]
                  tunnel: [w421] -> w342
                  tunnel: w341 -> [w413]
                  tunnel: w340 -> [w420]
                  tunnel: [w420] -> w339
                  tunnel: w338 -> [w419]
                  tunnel: [w419] -> w337
                  tunnel: w336 -> [w418]
                  tunnel: [w418] -> w335
                  tunnel: w334 -> [w415]
                  tunnel: w333 -> [w417]
                  tunnel: [w417] -> w332
                  tunnel: [w412] -> w331
                  tunnel: [w411] -> w330
                  tunnel: w346 -> [w442]
                  tunnel: w344 -> [w441]
                  tunnel: w342 -> [w443]
                  tunnel: [w440] -> w371
                  tunnel: [w448] -> w363
                  tunnel: w339 -> [w448]
                  tunnel: [w447] -> w361
                  tunnel: w337 -> [w447]
                  tunnel: [w446] -> w357
                  tunnel: w335 -> [w446]
                  tunnel: [w445] -> w352
                  tunnel: w332 -> [w445]
                  tunnel: [w435] -> w349
                  tunnel: [w441] -> w348
                  tunnel: w331 -> [w439]
                  tunnel: w330 -> [w438]
                  tunnel: [w449] -> w370
                  tunnel: [w456] -> w369
                  tunnel: w371 -> [w456]
                  tunnel: [w455] -> w364
                  tunnel: w363 -> [w455]
                  tunnel: [w454] -> w362
                  tunnel: w361 -> [w454]
                  tunnel: [w453] -> w358
                  tunnel: w357 -> [w453]
                  tunnel: [w452] -> w353
                  tunnel: w352 -> [w452]
                  tunnel: w349 -> [w451]
                  tunnel: w348 -> [w450]
                  tunnel: w370 -> [w478]
                  tunnel: w369 -> [w472]
                  tunnel: [w476] -> w365
                  tunnel: [w475] -> w350
                  tunnel: w364 -> [w475]
                  tunnel: w362 -> [w474]
                  tunnel: [w474] -> w360
                  tunnel: w358 -> [w473]
                  tunnel: [w471] -> w351
                  tunnel: w353 -> [w471]
                  frame #0 {
                    # "Time (s)"
                    # "Period (s)"
                    n85 = call <vilib>:"Read.vi"("Encoder Ref In"=w400) -> ("Counter Value"=w399:i32, "Encoder Ref Out"=w388:T30)  [unwired: 6 in, 3 out]
                    n86 = call <vilib>:"Read.vi"("AI Ref In"=w397) -> ("Values"=w396:dbl[], "AI Ref Out"=w387:T27)  [unwired: 8 in, 1 out]
                    n87 = Divide(x=w401, y=1000000) -> (x/y=w394:dbl)
                    n88 = Index Array(array=w396, index=0) -> (element=w373:dbl)
                    n89 = call "Tacho2Velocity_params.vi"() -> ("Cluster"=w375:T32)  [unwired: 5 in]
                    n90 = call "TF_Encoder2Position.vi"("Counter Value"=w399, "Offset"=0.0) -> ("Position [deg]"=w376:dbl)  [unwired: 3 in]
                    "Position Chart" <- w376
                    "Position [deg]" <- w376
                    n91 = call "TF_Tacho2Velocity.vi"("Tachometer Voltage [V]"=w373, "Tachometer param"=w375) -> ("Tachometer Velocity [deg/s]"=w374:dbl)  [unwired: 2 in]
                    n92 = call <vilib>:"Read.vi"("AI Ref In"=w378) -> ("Values"=w380:dbl[], "AI Ref Out"=w377:T27)  [unwired: 8 in, 1 out]
                    n93 = Index Array(array=w380, index=0) -> (element=w379:dbl)
                    n94 = flat-sequence {
                      tunnel: w394 -> [w408]
                      tunnel: [w405] -> w372
                      tunnel: w374 -> [w403]
                      frame #0 {
                        n95 = Reciprocal(x=w408) -> (1/x=w409:dbl)
                        n96 = call <vilib>:"Butterworth Filter PtByPt.vi"("order"=1, "filter type"=Filter_Passband_Type."Lowpass", "low cutoff freq: fl"=20.0, "sampling freq: fs"=w409, "x"=w403) -> ("Filtered x"=w405:dbl)  [unwired: 4 in, 1 out]
                      }
                    }
                    n97 = call "Tick Count2"() -> ("Tick Count(uSec)"=w393:u32)
                    n98 = Subtract(x=w393, y=w392) -> (x-y=w391:u32)
                    n99 = call "TF_MotorCurrentInput.vi"("Motor Current Monitor Value [V]"=w379) -> ("Current [A]"=→"Current [A]":dbl)
                    n100 = To Double Precision Float(number=w391) -> (double precision float=w390:dbl)
                    n101 = Divide(x=w390, y=1000000.0) -> (x/y=w385:dbl)
                    n102 = local write "Time (s)"(w385) -> ()
                    "Velocity Chart" <- w372
                    "Velocity [deg/s]" <- w372
                  }
                  frame #1 {
                    n103 = First Call?() -> (First Call?: T/F=w416:bool)
                    n104 = Or(x=w416, y=w415) -> (x .or. y?=w412:bool)
                    n105 = feedback #1() -> (w414:cluster{"time (s)":dbl, "setpoint":dbl}[])  [unwired: 1 in]
                    n106 = case shown="True" w412 {
                      tunnel: w413 -> [_ w427]
                      tunnel: [w423 w430] -> w411
                      tunnel: w414 -> [w423 _]
                      tunnel: w410 -> [_ w424]
                      frame False {
                      }
                      frame True {
                        n107 = Add(x=w424, y="Ramp Distance (°)") -> (x+y=w425:dbl)
                        n108 = call "TrajectoryRamp.vi"("Initial Time (s)"=w427, "Period (s)"=0.01, "Ramp Duration (s)"="Ramp Duration (s)", "Final Position (deg)"=w425, "Initial Position (deg)"=w424) -> ("Profile 2"=w430:cluster{"time (s)":dbl, "setpoint":dbl}[])  [unwired: 6 in]
                      }
                    }
                    n109 = feedback-in #1(w411) -> ()
                  }
                  frame #2 {
                    n110 = call <vilib>:"PID Setpoint Profile.vi"("reinitialize? (F)"=w439, "dt (s)"=w442, "setpoint profile"=w438) -> ("profile complete?"=w440:bool, "setpoint"=w436:dbl)  [unwired: 3 in, 2 out]
                    "Position Setpoint Chart" <- w436
                    "Position Setpoint [deg]" <- w436
                    n111 = call "ENPID.vi"("PID Settings"="PID Settings", "r"=w436, "y"=w441, "dy/dt"=w443, "dt (s)"=w442) -> (15:"u"=w435:dbl, 18:"u"=w437:cluster{"u":dbl, "up":dbl, "ui":dbl, "ud":dbl})  [unwired: 13 in]
                    "u_direct" <- w435
                    n112 = Unbundle By Name(w437) -> ("up"=→"up":dbl, "ui"=→"ui":dbl, "ud"=→"ud":dbl, "u"=→"u":dbl)
                  }
                  frame #3 {
                    w462 = 0.0  # [V]
                    w465 = 0.0  # [V]
                    w468 = -175.0  # [deg]
                    w469 = 175.0  # [deg]
                    w464 = -10.0  # [V]
                    w461 = 10.0  # [V]
                    # "Safety block"
                    n113 = call "TF_MotorCurrentOutput.vi"("Motor Current Setpoint [A]"=w451) -> ("Motor Current Setpoint [V]"=w470:dbl)
                    n114 = In Range and Coerce(upper limit=w461, x=w470, lower limit=w464) -> (coerced(x)=w458:dbl)  [unwired: 1 out]
                    n115 = Less Or Equal?(x=w450, y=w469) -> (x <= y?=w467:bool)
                    n116 = Greater Or Equal?(x=w450, y=w468) -> (x >= y?=w466:bool)
                    n117 = And(x=w467, y=w466) -> (x .and. y?=w463:bool)
                    n118 = Select(t=w464, s=w466, f=w465) -> (s? t:f=w460:dbl)
                    n119 = Select(t=w461, s=w463, f=w462) -> (s? t:f=w459:dbl)
                    n120 = In Range and Coerce(upper limit=w459, x=w458, lower limit=w460) -> (coerced(x)=w457:dbl)  [unwired: 1 out]
                    n121 = Select "Within Position Range?"(t=w458, s=w463, f=w457) -> (s? t:f=w449:dbl)
                    "Current Setpoint Chart" <- w449
                    "Current Setpoint [A]" <- w449
                  }
                  frame #4 {
                    # "Motor Current Setpoint"
                    n122 = Build Array(w478) -> (w477:dbl[])
                    n123 = call <vilib>:"Write.vi"("Values"=w477, "AO Ref In"=w473) -> ("AO Ref Out"=w476:T19)  [unwired: 7 in, 1 out]
                    n124 = case shown="True" w472 {
                      frame False {
                      }
                      frame True {
                        n125 = local write "Run"(FALSE) -> ()
                      }
                    }
                  }
                }
              }
            }
          }
          frame #2 {
          }
        }
        n126 = node-c288() -> ()  [unwired: 1 in, 1 out]
      }
      n127 = node-c288(w150) -> ()  [unwired: 1 out]
      n128 = node-c288(w157) -> ()  [unwired: 1 out]
      "Time (s)" <- 0.0
      "Running" <- 0.0 ("Running")
    }
    frame #5 {
      # "Tachometer"
      # "Motor Current Monitor"
      # "Motr Current Setpoint"
      # "Encoder"
      # "Close everything"
      n129 = call <vilib>:"Stop.vi"("Encoder Ref In"=w496) -> ("Encoder Ref Out"=w501:T30)  [unwired: 9 in, 1 out]
      n130 = Build Array(0.0) -> (w498:dbl[])
      n131 = call <vilib>:"Write.vi"("Values"=w498, "AO Ref In"=w497) -> ("AO Ref Out"=w500:T19)  [unwired: 7 in, 1 out]
      n132 = call <vilib>:"Close.vi"("AO Ref In"=w493) -> ()  [unwired: 10 in, 1 out]
      n133 = call <vilib>:"Close.vi"("Encoder Ref In"=w501) -> ()  [unwired: 10 in, 1 out]
      n134 = call <vilib>:"Close.vi"("AI Ref In"=w495) -> ()  [unwired: 10 in, 1 out]
      n135 = call <vilib>:"Close.vi"("AI Ref In"=w494) -> ()  [unwired: 10 in, 1 out]
      n136 = call <vilib>:"Close.vi"("AO Ref In"=w500) -> ()  [unwired: 10 in, 1 out]
    }
  }
